vi "UpdateConditions.vi"(6 "ConditionType":T3, 7 "dg_op":string, 8 "error in (no error)":errorcluster, 10 "conditions":T1[](array[typedef]), 11 "operating states in":variant) -> (0 "error out":errorcluster, 3 "operating states out":variant)   [LabVIEW 2017, in "Trigger.lvlib"]
uses:
  <vilib>/addons/InsightCM/Devices/Shared/Common/Trigger/Trigger.lvlib
  <vilib>/addons/InsightCM/Devices/Shared/Common/Trigger/controls/ConditionType.ctl
  <vilib>/addons/InsightCM/Devices/Shared/Common/Trigger/controls/TriggerCondition.ctl
  <vilib>/addons/InsightCM/MessageBus/Base/controls/Condition.ctl
  <vilib>/addons/InsightCM/Devices/Shared/Common/Trigger/controls/TriggerOperatingState.ctl
  <vilib>/addons/InsightCM/MessageBus/Base/controls/KeyValuePair.ctl
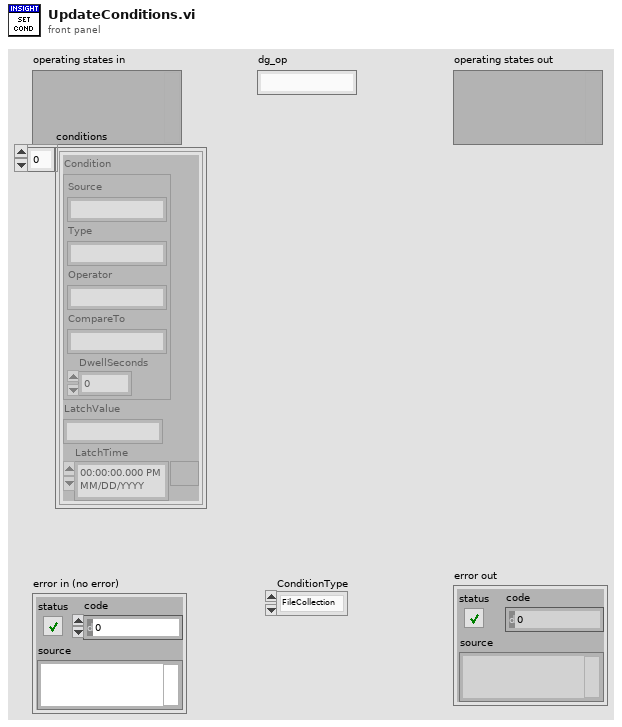
[diagram p1: front panel]
types:
  T1 = typedef "Trigger.lvlib/TriggerCondition.ctl" = cluster{"Condition":T2, "LatchValue":string, "LatchTime":timestamp}
  T2 = typedef "Condition.ctl" = cluster{"Source":string, "Type":string, "Operator":string, "CompareTo":string, "DwellSeconds":dbl}
  T3 = typedef "Trigger.lvlib/ConditionType.ctl" = enum16{"FileCollection", "TrendCollection"}
  T4 = typedef "Trigger.lvlib/TriggerOperatingState.ctl" = cluster{"Id":string, "Name":string, "Properties":T5[], "TrendExpression":string, "TrendConditions":T1[], "FileExpression":string, "FileConditions":T1[]}
  T5 = typedef "KeyValuePair.ctl" = cluster{"Key":string, "Value":string}
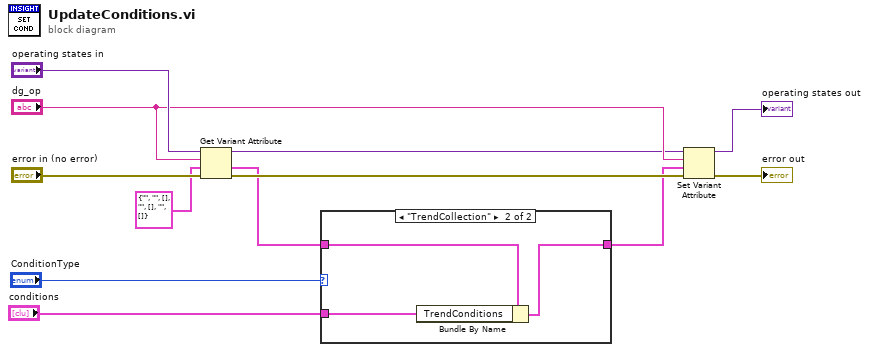
[diagram p0: block diagram]
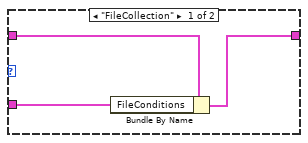
[diagram p2: hidden frame]
diagram:
  n1 = Get Variant Attribute(Variant="operating states in", name="dg_op", default value (empty Variant)=T4 {"Id"="", "Name"="", "Properties"=[], "TrendExpression"="", "TrendConditions"=[], "FileExpression"="", "FileConditions"=[]} ("OperatingState"), error in="error in (no error)") -> (duplicate Variant=w6:variant, value=w2:T4, error out=w9:errorcluster)  [unwired: 1 out]
  n2 = case shown="\"TrendCollection\"" "ConditionType" {
    tunnel: w2 -> [w15 w18]
    tunnel: [w14 w17] -> w1
    tunnel: "conditions" -> [w13 w16]
    frame "FileCollection" {
      n3 = Bundle By Name(cluster=w15, "FileConditions"=w13) -> (w14:T4)
    }
    frame "TrendCollection" {
      n4 = Bundle By Name(cluster=w18, "TrendConditions"=w16) -> (w17:T4)
    }
  }
  n5 = Set Variant Attribute(Variant=w6, name="dg_op", value=w1, error in=w9) -> (Variant out=→"operating states out":variant, error out=→"error out":errorcluster)  [unwired: 1 out]
